vi "Init MCL.vi"(8 "Error In":errorcluster, 11 "MCL Reference":refnum<vi>) -> (0 "Error Out":errorcluster)   [LabVIEW 2023, in "Error Manager.lvlib"]
doc: "Blank VI with error handling."
uses:
  Error Manager.lvlib
  <vilib>/Utility/miscctls.llb/LVRowAndColumnTypeDef.ctl
  <vilib>/Utility/miscctls.llb/LVRowAndColumnUnsignedTypeDef.ctl
panel:
  # "Input\nInputs to the VI"
  # "Development\nControls or indicators that are useful for development or testing, but which are not outputs of the VI."
  # "Output\nOutputs of the VI"
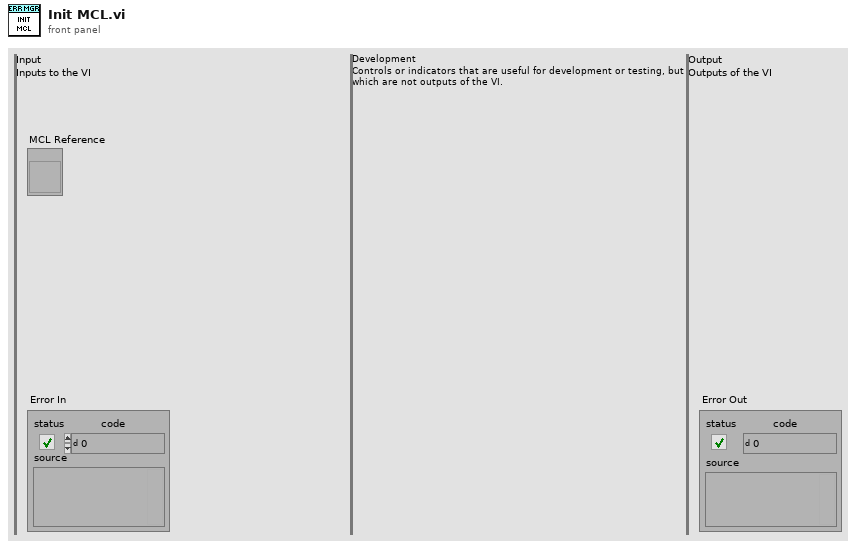
[diagram p1: front panel]
types:
  T1 = typedef "LVRowAndColumnUnsignedTypeDef.ctl" = cluster{"Row":u32, "Column":u32}
  T2 = typedef "LVRowAndColumnTypeDef.ctl" = cluster{"Row":i32, "Column":i32}
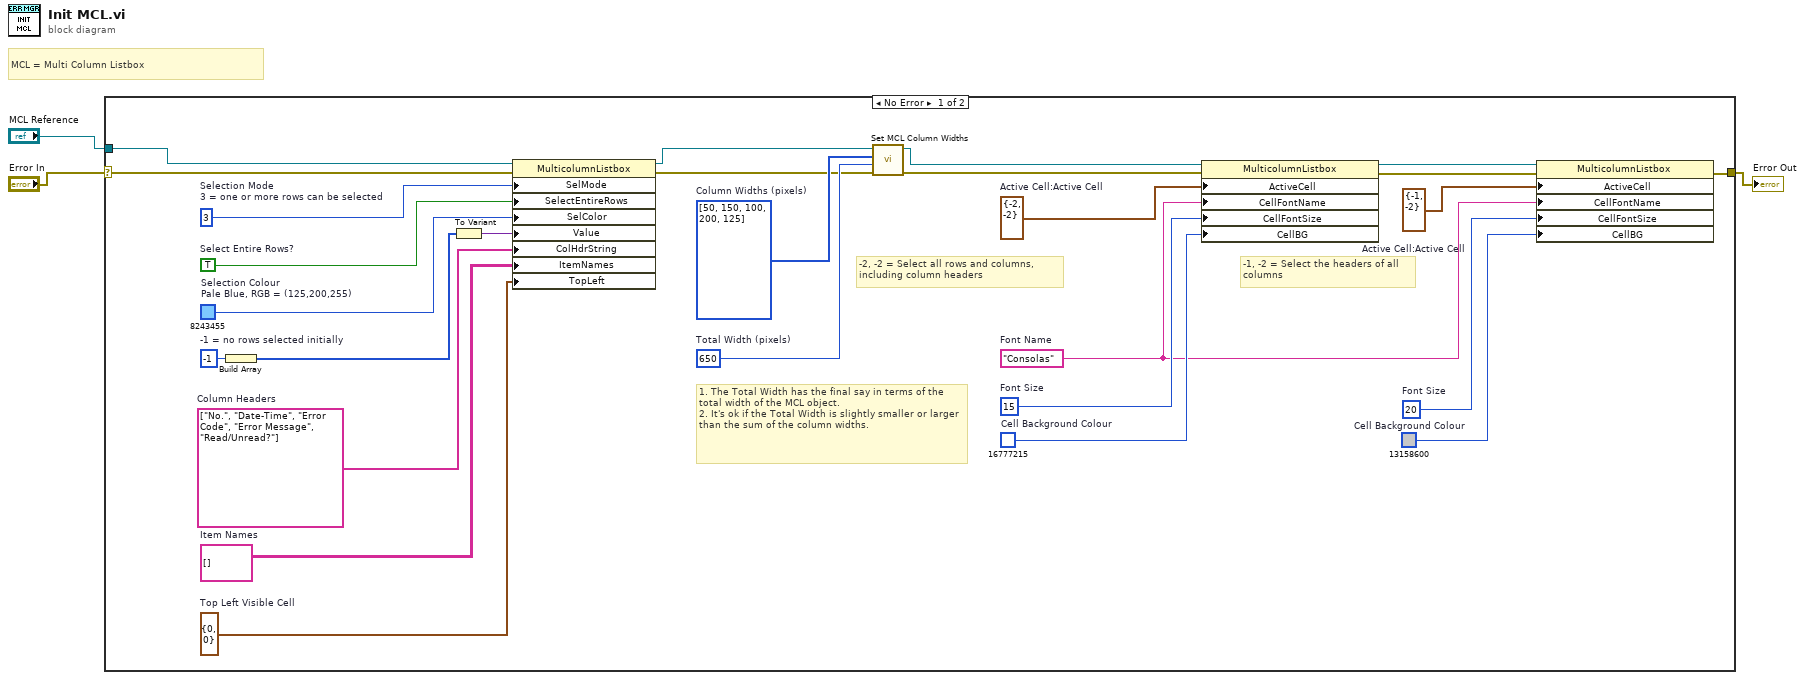
[diagram p0: block diagram]
diagram:
  # "MCL = Multi Column Listbox"
  n1 = case shown="No Error" "Error In" {
    selector: "Error In" -> [w30 w31]
    tunnel: "MCL Reference" -> [w12 _]
    tunnel: [w20 w31] -> w1
    frame No Error {
      w4 = T1 {"Row"=0, "Column"=0}  # Top Left Visible Cell
      w9 = -1  # -1 = no rows selected initially
      w10 = string[][] []  # Item Names
      w14 = 3  # Selection Mode 3 = one or more rows can be selected
      w5 = u32 8243455  # Selection Colour Pale Blue, RGB = (125,200,255)
      w6 = TRUE  # Select Entire Rows?
      w16 = u32 13158600  # Cell Background Colour
      w17 = u32 20  # Font Size
      w19 = T2 {"Row"=-1, "Column"=-2}  # Active Cell:Active Cell
      w23 = u32 16777215  # Cell Background Colour
      w24 = u32 15  # Font Size
      w18 = "Consolas"  # Font Name
      w25 = T2 {"Row"=-2, "Column"=-2}  # Active Cell:Active Cell
      w28 = u32 650  # Total Width (pixels)
      w29 = u32[] [50, 150, 100, 200, 125]  # Column Widths (pixels)
      w11 = string[] ["No.", "Date-Time", "Error Code", "Error Message", "Read/Unread?"]  # Column Headers
      # "-1, -2 = Select the headers of all columns"
      # "-2, -2 = Select all rows and columns, including column headers"
      # "1. The Total Width has the final say in terms of the total width of the MCL object.\n2. It's ok if the Total Width is slightly smaller or larger than the sum of the column widths."
      n2 = Build Array(w9) -> (w8:i32[])
      n3 = To Variant(anything=w8) -> (Variant=w7:variant)
      n4 = property class="MulticolumnListbox"(reference=w12, error in=w30, "SelMode"=w14, "SelectEntireRows"=w6, "SelColor"=w5, "Value"=w7, "ColHdrString"=w11, "ItemNames"=w10, "TopLeft"=w4) -> (reference out=w13:refnum<vi>, error out=w15:errorcluster)
      n5 = call "Set MCL Column Widths.vi"(8:w15, 9:w28, 10:w29, 11:w13) -> (0:w26:errorcluster, 3:w27:refnum<vi>)  [unwired: 6 in]
      n6 = property class="MulticolumnListbox"(reference=w27, error in=w26, "ActiveCell"=w25, "CellFontName"=w18, "CellFontSize"=w24, "CellBG"=w23) -> (reference out=w21:refnum<vi>, error out=w22:errorcluster)
      n7 = property class="MulticolumnListbox"(reference=w21, error in=w22, "ActiveCell"=w19, "CellFontName"=w18, "CellFontSize"=w17, "CellBG"=w16) -> (error out=w20:errorcluster)  [unwired: 1 out]
    }
    frame Error {
    }
  }
  "Error Out" <- w1
